vi "Write Outgoing Bytes.vi"(8 "error in (no error)":errorcluster, 9 "timeout (2000 ms)":i32=2000, 10 "Bytes":u8[](array[numeric]) format="%08b", 11 "WSConnection in":refnum<class "WebsocketsConnection.lvclass">) -> (0 "error out":errorcluster, 3 "WSConnection":refnum<class "WebsocketsConnection.lvclass">)   [LabVIEW 2013, in "MQTT_Websockets.lvlib" / "WebsocketsConnection.lvclass"]
uses:
  WebsocketsConnection.lvclass
  WebsocketsConnection.lvclass/WebsocketsConnection.ctl
  <vilib>/MediaMongrels Ltd/WebSockets/WebSockets/WebSocket/WebSocket.lvclass
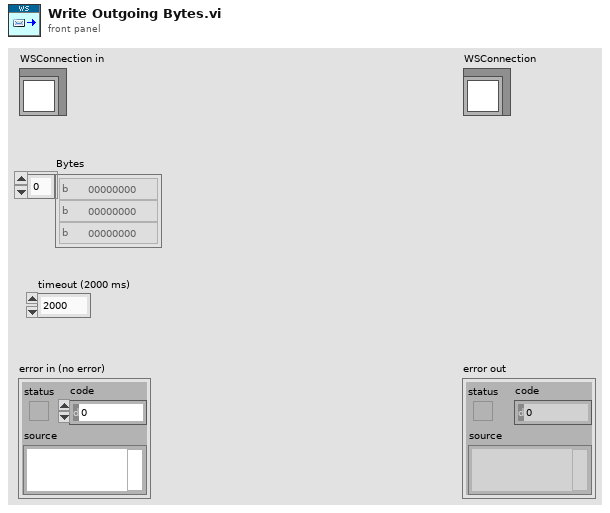
[diagram p1: front panel]
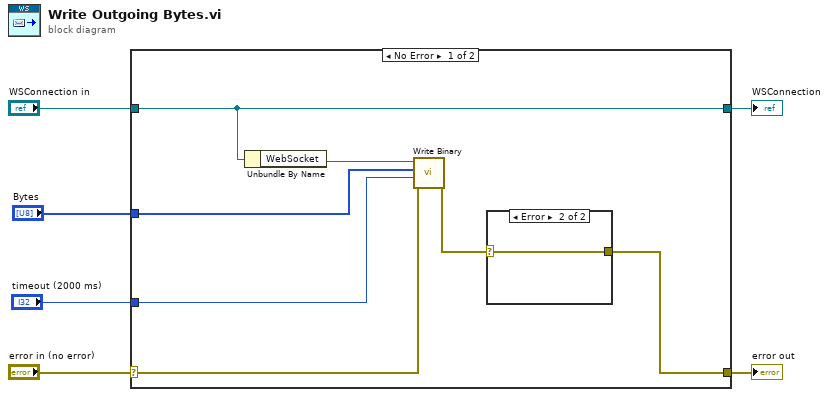
[diagram p0: block diagram]
diagram:
  n1 = case shown="No Error" "error in (no error)" {
    selector: "error in (no error)" -> [w10 w17]
    tunnel: [w13 w17] -> w5
    tunnel: [w8 w16] -> w3
    tunnel: "WSConnection in" -> [w8 w16]
    tunnel: "Bytes" -> [w11 _]
    tunnel: "timeout (2000 ms)" -> [w7 _]
    frame No Error {
      n2 = Unbundle By Name(w8) -> ("WebSocket"=w12:refnum<class "WebSocket.lvclass">)
      n3 = call-dynamic "Write Binary.vi"("error in (no error)"=w10, "timeout ms (5000)"=w7, "Binary Data"=w11, "WebSocket in"=w12) -> ("error out"=w9:errorcluster)  [unwired: 6 in, 1 out]
      n4 = case shown="Error" w9 {
        selector: w9 -> [w14 w15]
        tunnel: [w14 w15] -> w13
        frame No Error {
        }
        frame Error {
        }
      }
    }
    frame Error {
    }
  }
  "error out" <- w5
  "WSConnection" <- w3
